vi "SECoP-addPropertyString.vi"(8 "error in (no error)":errorcluster, 9 "property value":string, 10 "property name":string, 11 "DLL path (in)":T1) -> (0 "error out":errorcluster, 3 "DLL path (out)":T1)   [LabVIEW 2023, in "SECoP.lvlib"]
doc: "Call <b>\"SECoP-addPropertyString.vi\"</b> to append a SECoP string property to the last SEC node, module, command or parameter. This is a convenience function like \"SECoP-addProperty.vi\" with a string.\n\n<b>DLL path</b> input and output of cluster from \"SECoP-Initialize.vi\"\n<b>property name</b> name of property\n<b>property value</b> value of the property"
uses:
  SECoP.lvlib
  SECoP-libraries.ctl
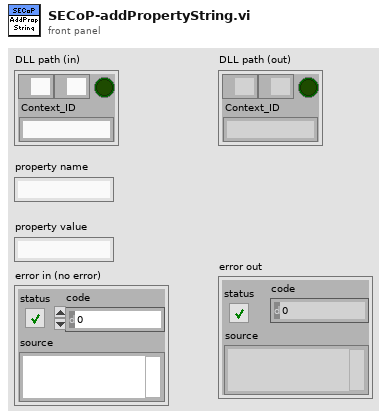
[diagram p1: front panel]
types:
  T1 = typedef "SECoP.lvlib/SECoP-libraries.ctl" = cluster{"serverDLL":path, "variantDLL":path, "cleanup_mode":bool, "Context_ID":string}
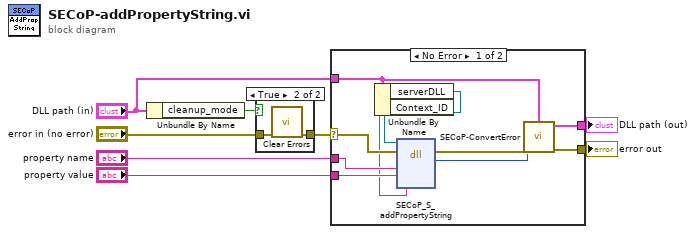
[diagram p0: block diagram]
diagram:
  n1 = Unbundle By Name("DLL path (in)") -> ("cleanup_mode"=w4:bool)
  n2 = case shown="True" w4 {
    tunnel: "error in (no error)" -> [w9 w11]
    tunnel: [w9 w10] -> w2
    frame False {
    }
    frame True {
      n3 = call <vilib>:"Clear Errors.vi"("error in (no error)"=w11) -> ("error out"=w10:errorcluster)  [unwired: 5 in, 1 out]
    }
  }
  n4 = case shown="No Error" w2 {
    selector: w2 -> [w19 w22]
    tunnel: "DLL path (in)" -> [w14 w23]
    tunnel: [w20 w23] -> w8
    tunnel: [w21 w22] -> w7
    tunnel: "property name" -> [w16 _]
    tunnel: "property value" -> [w15 _]
    frame No Error {
      n5 = Unbundle By Name(w14) -> ("serverDLL"=w13:path, "Context_ID"=w12:string)
      n6 = dll-call lib="C:/Users/user/Desktop/x86_64/SECoP64.dll" fn="SECoP_S_addPropertyString"(path in=w13, error in=w19, "name"=w16, "value"=w15, "szContextID"=w12) -> (error out=w18:errorcluster, "return type"=w17:i32)  [unwired: 4 in, 1 out]
      n7 = call "SECoP-ConvertError.vi"("return code"=w17, "error in (no error)"=w18, "DLL path (in)"=w14) -> ("error out"=w21:errorcluster, "DLL path (out)"=w20:T1)  [unwired: 7 in]
    }
    frame Error {
    }
  }
  "DLL path (out)" <- w8
  "error out" <- w7
